vi "Get Segment File Condition Caption.vi"(11 "Segment Files By":T1) -> (3 "Segment File Size Caption":string)   [LabVIEW 2020, in "AIM ARINC 664 System Explorer.lvlib" / "Implementation.lvlib"]
uses:
  System Explorer/Implementation/Implementation.lvlib
  FileSegmentType.ctl
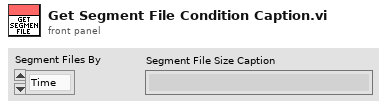
[diagram p1: front panel]
types:
  T1 = typedef "FileSegmentType.ctl" = enum16{"Time", "Size"}
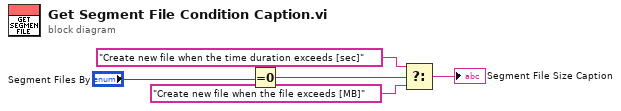
[diagram p0: block diagram]
diagram:
  n1 = Equal To 0?(x="Segment Files By") -> (x = 0?=w2:bool)
  n2 = Select(t="Create new file when the time duration exceeds [sec]" ("Caption.Text"), s=w2, f="Create new file when the file exceeds [MB]" ("Caption.Text")) -> (s? t:f=→"Segment File Size Caption":string)
